vi "TEST MMI Scaling (By Reference).vi"() -> ()   [LabVIEW 2021, in "IObject.lvclass"]
uses:
  IObject.lvclass
  Object/Object.lvclass
  C:/Projects/Dynamic-Scaling/Dynamic Scaling/IObject.lvclass
  IContainer/Viewport/Viewport.lvclass
  IContainer/Divider/Splitter/Splitter.lvclass
  Interaction By Refererence/Interaction By Refererence.lvclass
panel:
  out "XY Graph 6":cluster{"X":dbl, "Y":dbl}[](graph)
  out "XY Graph 5":cluster{"X":dbl, "Y":dbl}[](graph)
  out "XY Graph 4":cluster{"X":dbl, "Y":dbl}[](graph)
  out "XY Graph 3":cluster{"X":dbl, "Y":dbl}[](graph)
  out "XY Graph 2":cluster{"X":dbl, "Y":dbl}[](graph)
  out "XY Graph":cluster{"X":dbl, "Y":dbl}[](graph)
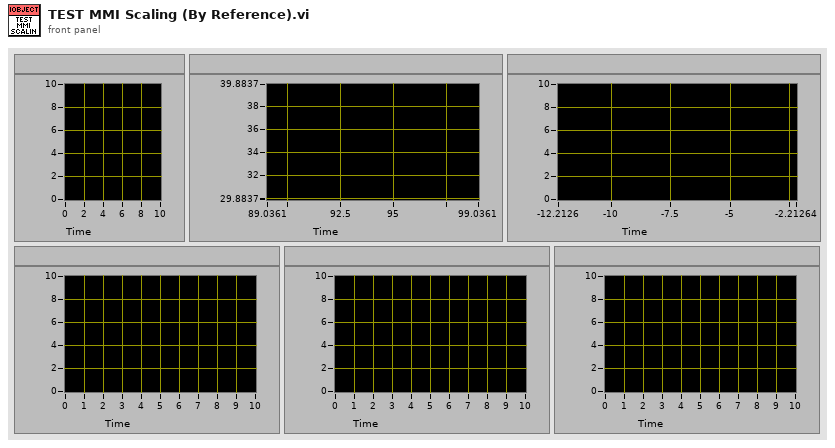
[diagram p1: front panel]
types:
  T1 = cluster{"Left":dbl, "Top":dbl, "Right":dbl, "Bottom":dbl}
  T2 = typedef "LVRectTypeDef.ctl" = cluster{"Left":i16, "Top":i16, "Right":i16, "Bottom":i16}
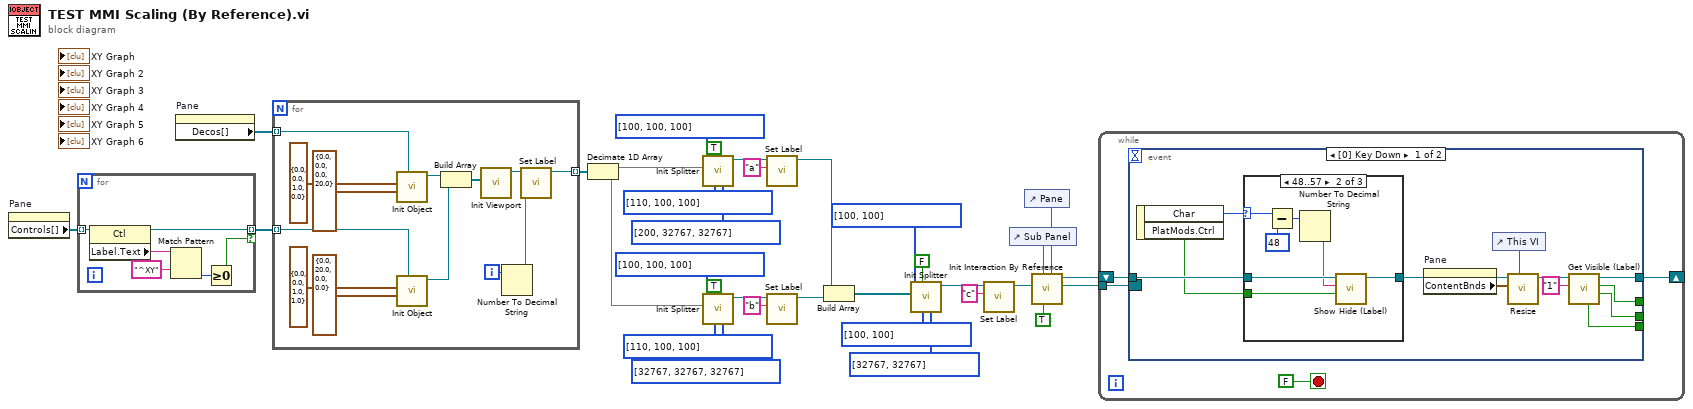
[diagram p0: block diagram]
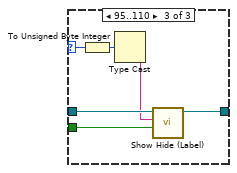
[diagram p3: hidden frame]
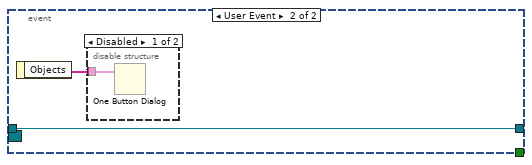
[diagram p4: hidden frame]
diagram:
  n1 = property on="Pane" class="Pane"() -> ("Controls[]"=w7:refnum<vi>[])  [unwired: 2 in, 2 out]
  n2 = for {
    tunnel: w7 -> [w39] mode=indexing
    tunnel: [w36] -> w6 mode=indexing if=w34
    n3 = property class="Ctl"(reference=w39) -> (reference out=w36:refnum<vi>, "Label.Text"=w38:string)  [unwired: 1 in, 1 out]
    n4 = Match Pattern(string=w38, regular expression="^XY") -> (offset past match=w35:i32)  [unwired: 1 in, 3 out]
    n5 = Greater Or Equal To 0?(x=w35) -> (x >= 0?=w34:bool)
  }
  n6 = property on="Pane" class="Pane"() -> ("Decos[]"=w31:refnum<vi>[])  [unwired: 2 in, 2 out]
  n7 = for {
    tunnel: w31 -> [w52] mode=indexing
    tunnel: [w41] -> w25 mode=indexing
    tunnel: w6 -> [w45] mode=indexing
    i -> [w51]
    n8 = call "Init Object.vi"("GObj Refnum"=w52, "B [0, 0, 0, 0]"=T1 {"Left"=0.0, "Top"=0.0, "Right"=0.0, "Bottom"=20.0} ("B"), "A [0, 0, 1, 1]"=T1 {"Left"=0.0, "Top"=0.0, "Right"=1.0, "Bottom"=0.0} ("A")) -> ("MMI Scaling out"=w43:refnum<class "Object.lvclass">)  [unwired: 7 in, 1 out]
    n9 = call "Init Object.vi"("GObj Refnum"=w45, "B [0, 0, 0, 0]"=T1 {"Left"=0.0, "Top"=20.0, "Right"=0.0, "Bottom"=0.0} ("B"), "A [0, 0, 1, 1]"=T1 {"Left"=0.0, "Top"=0.0, "Right"=1.0, "Bottom"=1.0} ("A")) -> ("MMI Scaling out"=w42:refnum<class "Object.lvclass">)  [unwired: 7 in, 1 out]
    n10 = Build Array(w43, w42) -> (w48:refnum<class "Object.lvclass">[])
    n11 = call "Init Viewport.vi"("Items"=w48) -> ("Viewport out"=w40:refnum<class "Viewport.lvclass">)  [unwired: 9 in, 1 out]
    n12 = Number To Decimal String(number=w51) -> (decimal integer string=w44:string)  [unwired: 1 in]
    n13 = call "Set Label.vi"("Label"=w44, "MMI Scaling in"=w40) -> ("MMI Scaling out"=w41:refnum<class "Viewport.lvclass">)  [unwired: 8 in, 1 out]
  }
  n14 = Decimate 1D Array(w25) -> (w26:refnum<class "Viewport.lvclass">[], w18:refnum<class "Viewport.lvclass">[])
  n15 = call "Init Splitter.vi"("Maximal size"=i16[] [200, 32767, 32767] ("Minimal size"), "Minimal size"=i16[] [110, 100, 100], "Vertical? [F, hor.]"=TRUE, "Relative size"=i16[] [100, 100, 100] ("Minimal size"), "Items"=w26) -> ("Splitter out"=w33:refnum<class "Splitter.lvclass">)  [unwired: 5 in, 1 out]
  n16 = call "Init Splitter.vi"("Maximal size"=i16[] [32767, 32767, 32767] ("Minimal size"), "Minimal size"=i16[] [110, 100, 100], "Vertical? [F, hor.]"=TRUE, "Relative size"=i16[] [100, 100, 100] ("Minimal size"), "Items"=w18) -> ("Splitter out"=w19:refnum<class "Splitter.lvclass">)  [unwired: 5 in, 1 out]
  n17 = call "Set Label.vi"("Label"="a", "MMI Scaling in"=w33) -> ("MMI Scaling out"=w15:refnum<class "Splitter.lvclass">)  [unwired: 8 in, 1 out]
  n18 = call "Set Label.vi"("Label"="b", "MMI Scaling in"=w19) -> ("MMI Scaling out"=w17:refnum<class "Splitter.lvclass">)  [unwired: 8 in, 1 out]
  n19 = Build Array(w15, w17) -> (w16:refnum<class "Splitter.lvclass">[])
  n20 = call "Init Splitter.vi"("Maximal size"=i16[] [32767, 32767] ("Size"), "Minimal size"=i16[] [100, 100] ("Size"), "Vertical? [F, hor.]"=FALSE, "Relative size"=i16[] [100, 100] ("Size"), "Items"=w16) -> ("Splitter out"=w9:refnum<class "Splitter.lvclass">)  [unwired: 5 in, 1 out]
  n21 = call "Set Label.vi"("Label"="c", "MMI Scaling in"=w9) -> ("MMI Scaling out"=w8:refnum<class "Splitter.lvclass">)  [unwired: 8 in, 1 out]
  n22 = control-ref of="Sub Panel"() -> (w5:refnum<vi>)
  n23 = control-ref of="Pane"() -> (w3:refnum<vi>)
  n24 = call "Init Interaction By Reference.vi"("Pane"=w3, "Register resize events? [F]"=TRUE, "Sub Panel"=w5, "IObject"=w8) -> ("Object resize event"=w2:refnum<event-registration>, "Interaction out"=w4:refnum<class "Interaction By Refererence.lvclass">)  [unwired: 5 in, 1 out]
  n25 = while {
    shift-right: [w54] -> _
    shift-left: w4 -> [w56]
    tunnel: w2 -> [w53]
    stop <- FALSE stop-if-true
    n26 = event shown="[0] Key Down" {
      selector: w53 -> [_ _]
      dyn-events: _ -> [_ _]
      timeout: _ -> [_ _]
      tunnel: w56 -> [w64 w84]
      tunnel: [w61 w84] -> w54
      tunnel: [w59 _] -> _
      tunnel: [w58 _] -> _
      tunnel: [w57 _] -> _
      event Key Down {
        n27 = event-data() -> ("Char"=w66:i16, "PlatMods.Ctrl"=w63:bool)  [unwired: 1 in]
        n28 = case shown="48..57" w66 {
          selector: w66 -> [_ w76 w80]
          tunnel: [w69 w72 w81] -> w65
          tunnel: w64 -> [w69 w74 w82]
          tunnel: w63 -> [_ w71 w78]
          frame Default {
          }
          frame 48..57 {
            n29 = Subtract(x=w76, y=i16 48) -> (x-y=w73:i16)
            n30 = Number To Decimal String(number=w73) -> (decimal integer string=w70:string)  [unwired: 1 in]
            n31 = call-dynamic "Show Hide (Label).vi"("Show? [T]"=w71, "Label"=w70, "MMI Scaling in"=w74) -> ("MMI Scaling out"=w72:refnum<class "Interaction By Refererence.lvclass">)  [unwired: 6 in, 2 out]
          }
          frame 95..110 {
            n32 = To Unsigned Byte Integer(number=w80) -> (unsigned 8bit integer=w79:u8)
            n33 = Type Cast(x=w79) -> (*(type *) &x=w77:string)  [unwired: 1 in]
            n34 = call-dynamic "Show Hide (Label).vi"("Show? [T]"=w78, "Label"=w77, "MMI Scaling in"=w82) -> ("MMI Scaling out"=w81:refnum<class "Interaction By Refererence.lvclass">)  [unwired: 6 in, 2 out]
          }
        }
        n35 = property on="Pane" class="Pane"() -> ("ContentBnds"=w68:T2)  [unwired: 2 in, 2 out]
        n36 = control-ref of="This VI"() -> (w67:refnum<vi>)
        n37 = call-dynamic "Resize.vi"("VI Refnum"=w67, "Bounds"=w68, "MMI Scaling in"=w65) -> ("MMI Scaling out"=w62:refnum<class "Interaction By Refererence.lvclass">)  [unwired: 6 in, 2 out]
        n38 = call-dynamic "Get Visible (Label).vi"("Label"="1", "Interaction By Refererence in"=w62) -> ("Match?"=w58:bool, "Visible?"=w59:bool, "Interaction By Refererence out"=w61:refnum<class "Interaction By Refererence.lvclass">, "Item visible?"=w57:bool)  [unwired: 5 in, 1 out]
      }
      event User Event {
        n39 = event-data() -> ("Objects"=w83:string[])  [unwired: 1 in]
        n40 = disable-structure shown="Disabled" {
          disable-tunnel: w83 -> [w85 _]
          frame Disabled {
            n41 = One Button Dialog(message=w85) -> ()  [unwired: 1 in, 1 out]
          }
          frame Enabled {
          }
        }
      }
    }
  }
